vi "Round Time Down.vi"(11 "clock time":dbl format="%<%H:%M:%S>t") -> (3 "lower minute":dbl format="%<%H:%M:%S>t")   [LabVIEW 2019, in "Pet Feeder.lvlib"]
uses:
  Pet Feeder.lvlib
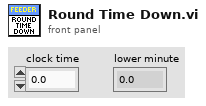
[diagram p1: front panel]
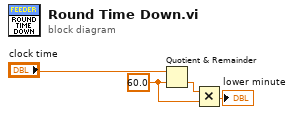
[diagram p0: block diagram]
diagram:
  w3 = 60.0 ("y")
  n1 = Quotient & Remainder(x="clock time", y=w3) -> (floor(x/y)=w2:dbl)  [unwired: 1 out]
  n2 = Multiply(x=w2, y=w3) -> (x*y=→"lower minute":dbl)
